vi "Set Color Ref.vi"(8 "error in (no error)":errorcluster caption="错误输入（无错误）", 10 "Color":refnum<k24>, 11 "Color输入":refnum<class "Color.lvclass">) -> (0 "error out":errorcluster caption="错误输出", 3 "Color输出":refnum<class "Color.lvclass">)   [LabVIEW 2012, in "Color.lvclass"]
uses:
  Color.lvclass
  System.Drawing
  Color.lvclass/Color.ctl
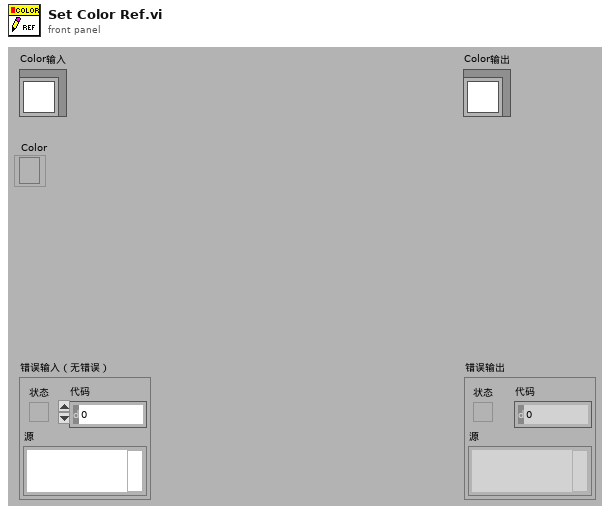
[diagram p1: front panel]
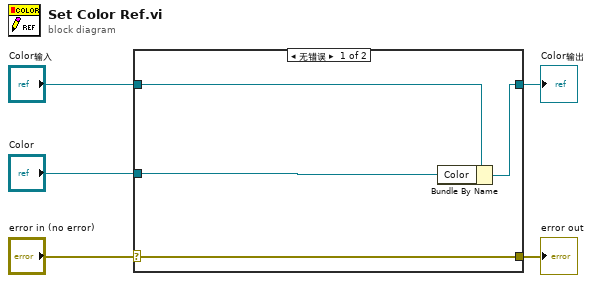
[diagram p0: block diagram]
diagram:
  n1 = case shown="无错误" "error in (no error)" {
    selector: "error in (no error)" -> [w9 w10]
    tunnel: [w9 w10] -> w4
    tunnel: [w7 w11] -> w2
    tunnel: "Color输入" -> [w8 w11]
    tunnel: "Color" -> [w6 _]
    frame No Error {
      n2 = Bundle By Name(cluster=w8, "Color"=w6) -> (w7:refnum<class "Color.lvclass">)
    }
    frame Error {
    }
  }
  "error out" <- w4
  "Color输出" <- w2
